vi "TxData_Organization_EVM_Selection_EIRP_only.vi"() -> ()   [LabVIEW 2023, in "ParsingData.lvlib"]
uses:
  <vilib>/Utility/file.llb/Read Delimited Spreadsheet (string).vi
  <vilib>/Utility/file.llb/Read Delimited Spreadsheet (DBL).vi
  ParsingData.lvlib
panel:
  in  "EVM?":dbl=-30.0 format="%#_13g"
  in  "EIRP_res":dbl=10.0
  in  "EIRP_Max":dbl=60.0
  in  "EIRP_Min":dbl=-10.0
  in  "CalPower ¸ÉÀv":dbl=70.0 format="%#_13g"
  in  "Input power_res":dbl=5.0
  in  "Input power_up":dbl=-20.0
  in  "Input power_low":dbl=-60.0
  out "Maximum_EIRP":T1 caption="Maximum EIRP"
  out "Minimum_EIRP":T1 caption="Minimum EIRP"
  out "Best EVM with EIRP steps":T2(array[cluster])
  in  "File Path":path=path "D:/_Project/_Code/LabVIEW/L_og_Backup/Cindy_20250224_litepoint_UD0630_one_panel"
  out "Max EVM : Mode             Polarity                     UD att                BFIC COM att           BFIC ele att                SG Power                      EIRP                           EVM":string[](array[string])
  out "EVM to EIRP":cluster{dbl[], "all rows":dbl[]}[](graph)
  # "X:EIRP        Y:EVM"
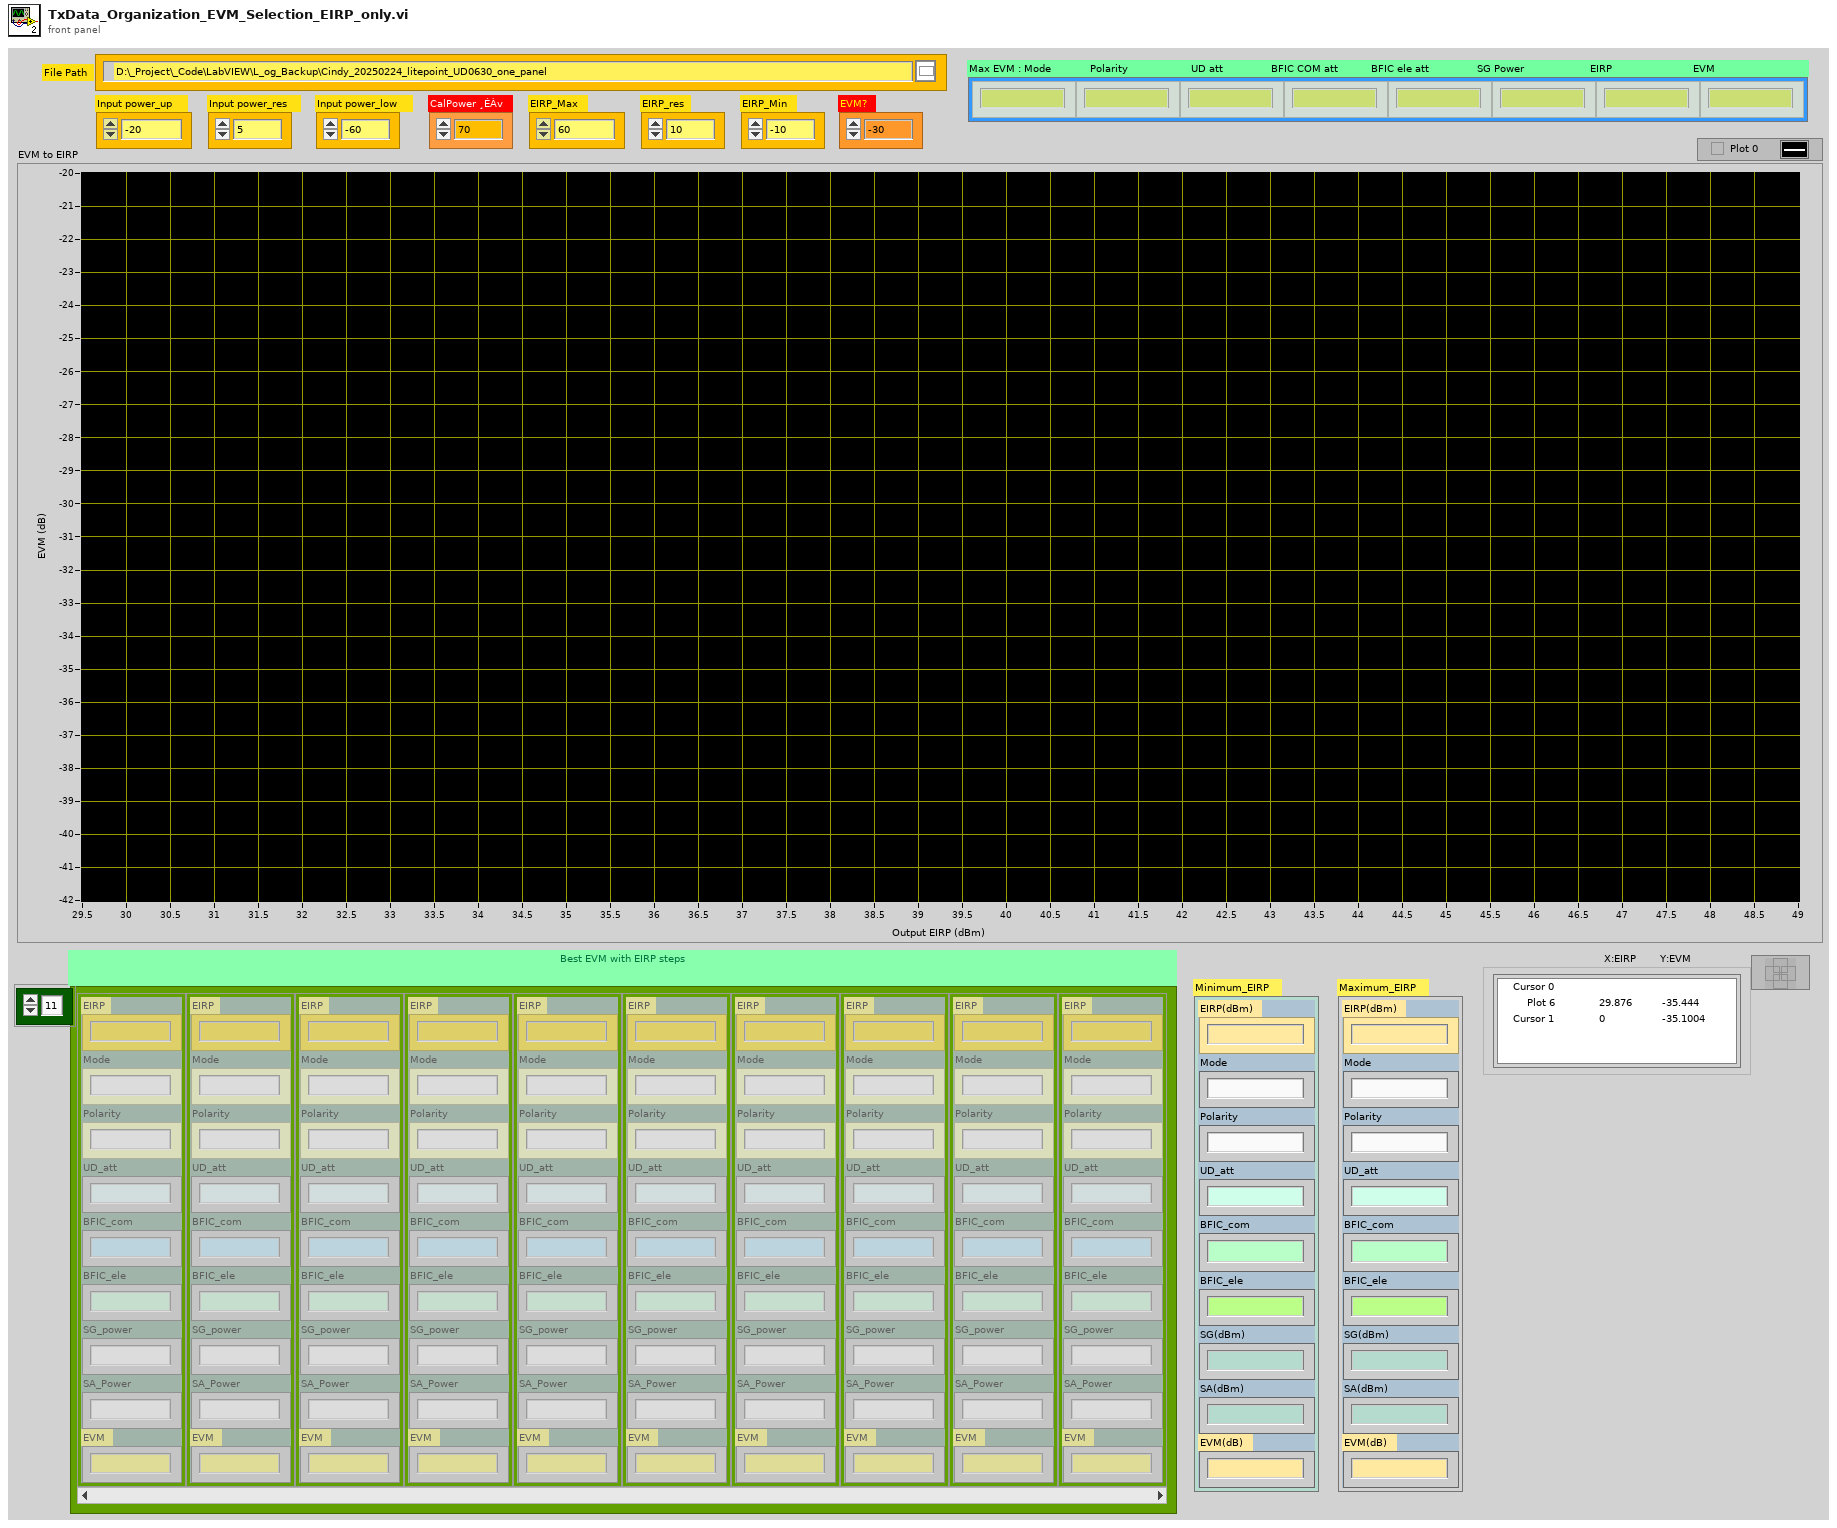
[diagram p1: front panel]
types:
  T1 = cluster{"EIRP(dBm)":string, "Mode":string, "Polarity":string, "UD_att":string, "BFIC_com":string, "BFIC_ele":string, "SG(dBm)":string, "SA(dBm)":string, "EVM(dB)":string}
  T2 = cluster{"EIRP":string, "Mode":string, "Polarity":string, "UD_att":string, "BFIC_com":string, "BFIC_ele":string, "SG_power":string, "SA_Power":string, "EVM":string}[]
  T3 = cluster{"[0]":string, "[1]":string, "[2]":string, "[3]":string, "[4]":string, "[5]":string, "[6]":string, "[7]":string, "[8]":string}
  T4 = cluster{"[0]":string, "[1]":string, "[2]":string, "[3]":string, "[4]":string, "[5]":string, "[6]":string, "[7]":string, "[8]":string}[]
  T5 = cluster{"EIRP":string, "Mode":string, "Polarity":string, "UD_att":string, "BFIC_com":string, "BFIC_ele":string, "SG_power":string, "SA_Power":string, "EVM":string}
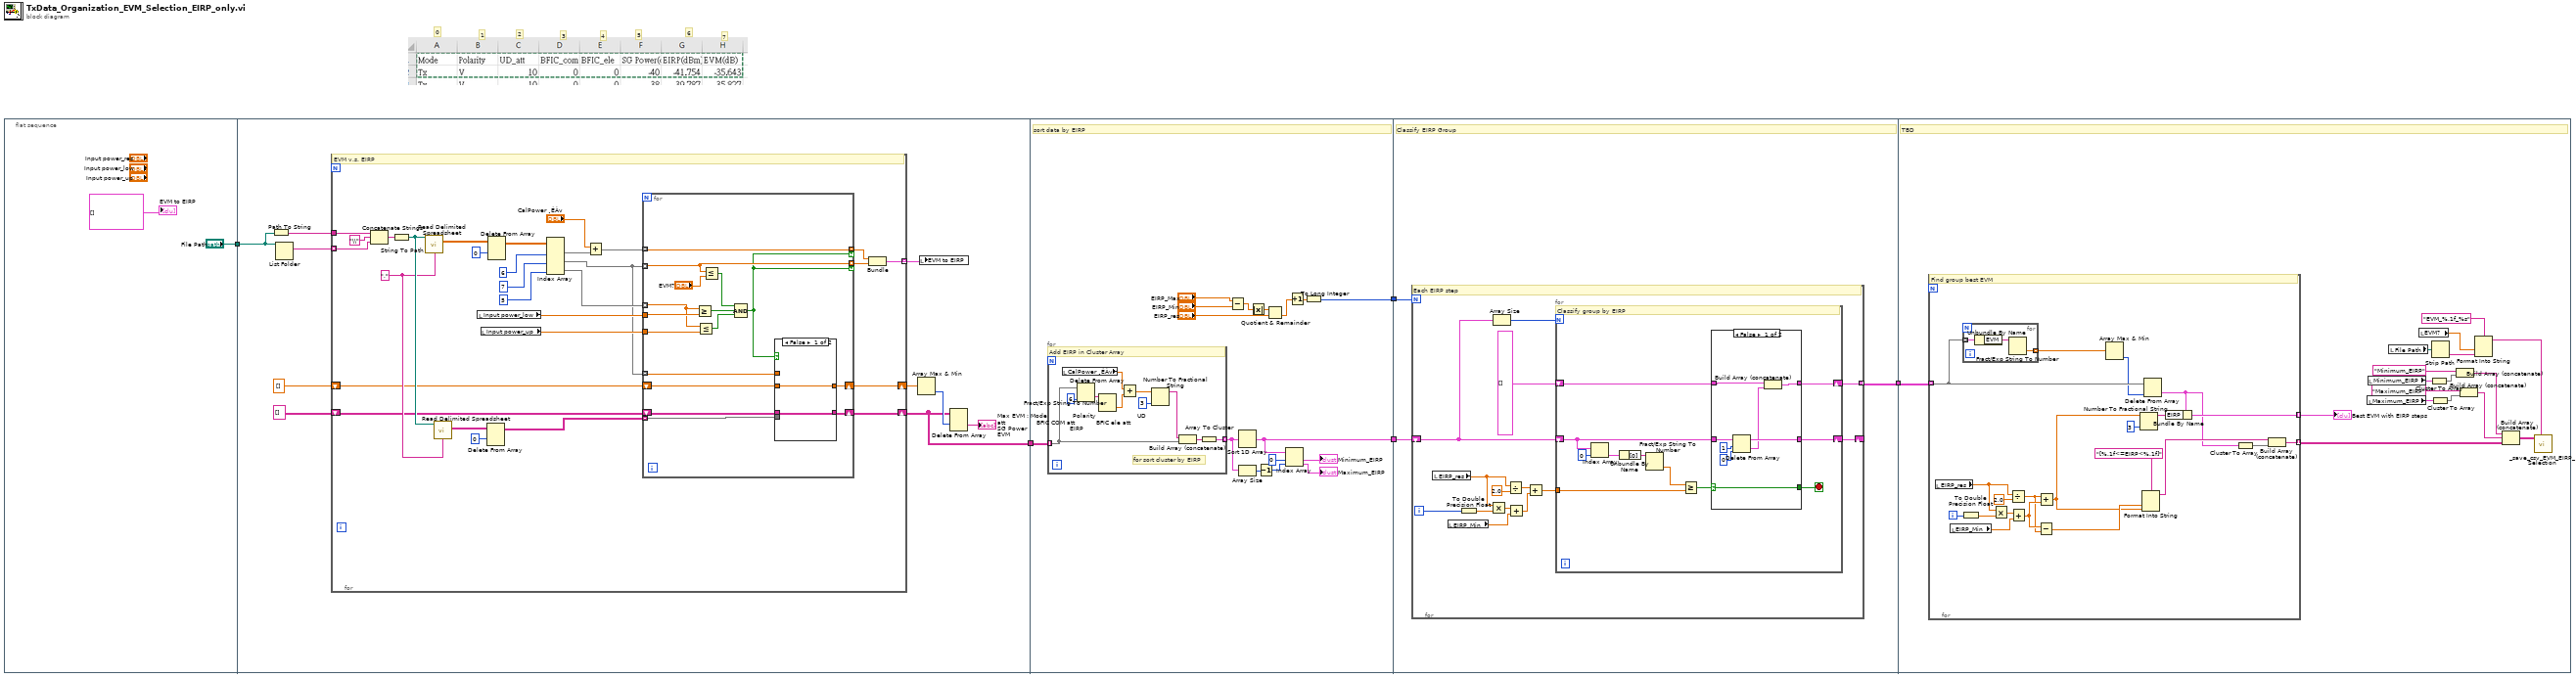
[diagram p0: block diagram]
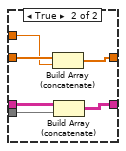
[diagram p2: hidden frame]
diagram:
  # "7"
  # "6"
  # "5"
  # "4"
  # "3"
  # "2"
  # "1"
  # "0"
  n1 = flat-sequence {
    tunnel: ["File Path"] -> w5
    tunnel: [w8] -> w1
    tunnel: w5 -> [w11]
    tunnel: w1 -> [w78]
    tunnel: [w76] -> w4
    tunnel: [w82] -> w3
    tunnel: w4 -> [w98]
    tunnel: w3 -> [w99]
    tunnel: [w97] -> w2
    tunnel: w2 -> [w152]
    frame #0 {
      "EVM to EIRP" <- cluster{dbl[], dbl[]}[] []
    }
    frame #1 {
      n2 = Path To String(path=w11) -> (string=w16:string)
      n3 = List Folder(path=w11) -> (filenames=w17:string[])  [unwired: 3 in, 3 out]
      n4 = for {
        tunnel: w17 -> [w44] mode=indexing
        tunnel: w16 -> [w46]
        tunnel: [w36] -> w9 mode=indexing
        shift-right: [w18] -> w8
        shift-left: string[][] [] -> [w22]
        shift-right: [w19] -> w14
        shift-left: dbl[] [] -> [w23]
        w27 = "," ("delimiter (\\t)")
        # "EVM v.s. EIRP"
        n5 = Concatenate Strings(w46, "\\" ("string"), w44) -> (w45:string)
        n6 = String To Path(string=w45) -> (path=w28:path)
        n7 = call-poly <vilib>:"Read Delimited Spreadsheet.vi"("file path (dialog if empty)"=w28, "delimiter (\\t)"=w27) -> ("all rows"=w42:dbl[][])  [unwired: 8 in, 5 out]
        n8 = call-poly <vilib>:"Read Delimited Spreadsheet.vi"("file path (dialog if empty)"=w28, "delimiter (\\t)"=w27) -> ("all rows"=w29:string[][])  [unwired: 8 in, 5 out]
        n9 = local read "Input power_low"() -> (w25:dbl)
        n10 = local read "Input power_up"() -> (w24:dbl)
        n11 = Delete From Array(array=w29, index (row)=0 ("disabled index (col)")) -> (array with subset deleted=w20:string[][])  [unwired: 2 in, 1 out]
        n12 = Delete From Array(array=w42, index (row)=0 ("disabled index (col)")) -> (array with subset deleted=w40:dbl[][])  [unwired: 2 in, 1 out]
        n13 = Index Array(array=w40, index (col) #1=6 ("disabled index (col)"), index (col) #2=7 ("index (col)"), index (col) #3=5 ("index (col)")) -> (element #1=w26:dbl[], element #2=w21:dbl[], element #3=w31:dbl[])  [unwired: 3 in]
        n14 = Add(x="CalPower ¸ÉÀv", y=w26) -> (x+y=w35:dbl[])
        n15 = for {
          tunnel: w35 -> [w60] mode=indexing
          tunnel: w21 -> [w61] mode=indexing
          tunnel: [w61] -> w33 mode=indexing if=w47
          tunnel: [w60] -> w34 mode=indexing if=w47
          tunnel: w31 -> [w58] mode=indexing
          tunnel: w25 -> [w59]
          tunnel: w24 -> [w57]
          shift-right: [w48] -> w19
          shift-left: w23 -> [w53]
          shift-right: [w49] -> w18
          shift-left: w22 -> [w51]
          tunnel: w21 -> [w52] mode=indexing
          tunnel: w20 -> [w50] mode=indexing
          n16 = Greater Or Equal?(x=w58, y=w59) -> (x >= y?=w55:bool)
          n17 = Less Or Equal?(x=w58, y=w57) -> (x <= y?=w56:bool)
          n18 = Less Or Equal?(x=w61, y="EVM?") -> (x <= y?=w54:bool)
          n19 = Compound Arithmetic op=AND(w54, w55, w56) -> (w47:bool)
          n20 = case shown="False" w47 {
            tunnel: w53 -> [w64 w70]
            tunnel: w52 -> [_ w69]
            tunnel: w51 -> [w63 w68]
            tunnel: w50 -> [_ w67]
            tunnel: [w63 w66] -> w49
            tunnel: [w64 w65] -> w48
            frame False {
            }
            frame True {
              n21 = Build Array (concatenate)(w70, w69) -> (w65:dbl[])
              n22 = Build Array (concatenate)(w68, w67) -> (w66:string[][])
            }
          }
        }
        n23 = Bundle(w34, w33) -> (w36:cluster{dbl[], dbl[]})  [unwired: 1 in]
      }
      n24 = Array Max & Min(array=w14) -> (min index (indices)=w13:i32)  [unwired: 3 out]
      n25 = local write "EVM to EIRP"(w9) -> ()
      n26 = Delete From Array(array=w8, index (row)=w13) -> (deleted portion=→"Max EVM : Mode             Polarity                     UD att                BFIC COM att           BFIC ele att                SG Power                      EIRP                           EVM":string[])  [unwired: 2 in, 1 out]
    }
    frame #2 {
      # "sort data by EIRP"
      n27 = for {
        tunnel: w78 -> [w87] mode=indexing
        tunnel: [w96] -> w77 mode=indexing
        # "for sort cluster by EIRP"
        # "Add EIRP in Cluster Array"
        n28 = local read "CalPower ¸ÉÀv"() -> (w90:dbl)
        n29 = Delete From Array(array=w87, index=6) -> (deleted portion=w93:string)  [unwired: 1 in, 1 out]
        n30 = Fract/Exp String To Number(string=w93) -> (number=w91:dbl)  [unwired: 3 in, 1 out]
        n31 = Add(x=w90, y=w91) -> (x+y=w92:dbl)
        n32 = Number To Fractional String(number=w92, precision (6)=i16 3) -> (F-format string=w89:string)  [unwired: 2 in]
        n33 = Build Array (concatenate)(w89, w87) -> (w94:string[])
        n34 = Array To Cluster(array=w94) -> (cluster=w96:T3)
      }
      n35 = Subtract(x="EIRP_Max", y="EIRP_Min") -> (x-y=w86:dbl)
      n36 = Sort 1D Array(array=w77) -> (sorted array=w76:T4)
      n37 = Array Size(array=w77) -> (size(s)=w75:i32)
      n38 = Absolute Value(x=w86) -> (abs(x)=w84:dbl)
      n39 = Decrement(x=w75) -> (x-1=w74:i32)
      n40 = Quotient & Remainder(x=w84, y="EIRP_res") -> (floor(x/y)=w85:dbl)  [unwired: 1 out]
      n41 = Index Array(array=w76, index #1=0 ("index"), index #2=w74) -> (element #1=→"Minimum_EIRP":T3, element #2=→"Maximum_EIRP":T3)
      n42 = Increment(x=w85) -> (x+1=w83:dbl)
      n43 = To Long Integer(number=w83) -> (32bit integer=w82:i32)
    }
    frame #3 {
      # "Classify EIRP Group"
      n44 = for {
        N: w99 -> [_]
        shift-right: [w104] -> _
        shift-left: w98 -> [w101]
        tunnel: [w103] -> w97 mode=indexing
        i -> [w109]
        # "Each EIRP step"
        n45 = local read "EIRP_res"() -> (w108:dbl)
        n46 = local read "EIRP_Min"() -> (w106:dbl)
        n47 = To Double Precision Float(number=w109) -> (double precision float=w107:dbl)
        n48 = Multiply(x=w108, y=w107) -> (x*y=w111:dbl)
        n49 = Array Size(array=w101) -> (size(s)=w102:i32)
        n50 = Divide(x=w108, y=2.0) -> (x/y=w112:dbl)
        n51 = Add(x=w111, y=w106) -> (x+y=w113:dbl)
        n52 = Add(x=w112, y=w113) -> (x+y=w105:dbl)
        n53 = for {
          N: w102 -> [_]
          tunnel: w105 -> [w120]
          shift-right: [w114] -> w104
          shift-left: w101 -> [w118]
          shift-right: [w116] -> w103
          shift-left: T2 [] ("reversed array") -> [w117]
          stop <- w115 stop-if-true
          # "Classify group by EIRP"
          n54 = Index Array(array=w118, index=0) -> (element=w124:T3)
          n55 = Unbundle By Name(w124) -> ("[0]"=w121:string)
          n56 = Fract/Exp String To Number(string=w121) -> (number=w122:dbl)  [unwired: 3 in, 1 out]
          n57 = Greater Or Equal?(x=w122, y=w120) -> (x >= y?=w119:bool)
          n58 = case shown="False" w119 {
            selector: w119 -> [w128 w135]
            tunnel: [w128 w135] -> w115
            tunnel: w118 -> [w132 w134]
            tunnel: [w129 w134] -> w114
            tunnel: w117 -> [w127 w133]
            tunnel: [w126 w133] -> w116
            frame False {
              n59 = Delete From Array(array=w132, length=1, index=0) -> (deleted portion=w125:T4, array with subset deleted=w129:T4)
              n60 = Build Array (concatenate)(w127, w125) -> (w126:T4)
            }
            frame True {
            }
          }
        }
      }
    }
    frame #4 {
      # "TBD"
      n61 = for {
        tunnel: w152 -> [w172] mode=indexing
        tunnel: [w154] -> w151 mode=indexing
        tunnel: [w167] -> w148 mode=indexing
        i -> [w161]
        # "Find group best EVM"
        n62 = local read "EIRP_res"() -> (w164:dbl)
        n63 = local read "EIRP_Min"() -> (w166:dbl)
        n64 = To Double Precision Float(number=w161) -> (double precision float=w165:dbl)
        n65 = for {
          tunnel: w172 -> [w176] mode=indexing
          tunnel: [w174] -> w173 mode=indexing
          n66 = Unbundle By Name(w176) -> ("EVM"=w175:string)
          n67 = Fract/Exp String To Number(string=w175) -> (number=w174:dbl)  [unwired: 3 in, 1 out]
        }
        n68 = Multiply(x=w164, y=w165) -> (x*y=w162:dbl)
        n69 = Divide(x=w164, y=2.0) -> (x/y=w159:dbl)
        n70 = Add(x=w162, y=w166) -> (x+y=w160:dbl)
        n71 = Subtract(x=w160, y=w159) -> (x-y=w157:dbl)
        n72 = Add(x=w159, y=w160) -> (x+y=w155:dbl)
        n73 = Array Max & Min(array=w173) -> (min index (indices)=w171:i32)  [unwired: 3 out]
        n74 = Number To Fractional String(number=w155, precision (6)=i16 3) -> (F-format string=w168:string)  [unwired: 2 in]
        n75 = Format Into String(format string="[%.1f<=EIRP<%.1f]", w157, w155) -> (resulting string=w156:string)  [unwired: 2 in, 1 out]
        n76 = Delete From Array(array=w172, index=w171) -> (deleted portion=w153:T5)  [unwired: 1 in, 1 out]
        n77 = Bundle By Name(cluster=w153, "EIRP"=w168) -> (w154:T5)
        n78 = Cluster To Array(cluster=w153) -> (array=w169:string[])
        n79 = Build Array (concatenate)(w156, w169) -> (w167:string[])
      }
      "Best EVM with EIRP steps" <- w151
      n80 = local read "Maximum_EIRP"() -> (w143:T1)
      n81 = local read "Minimum_EIRP"() -> (w146:T1)
      n82 = local read "File Path"() -> (w150:path)
      n83 = local read "EVM?"() -> (w138:dbl)
      n84 = Cluster To Array(cluster=w146) -> (array=w145:string[])
      n85 = Strip Path(path=w150) -> (name=w137:string)  [unwired: 1 out]
      n86 = Cluster To Array(cluster=w143) -> (array=w142:string[])
      n87 = Build Array (concatenate)("Minimum_EIRP" ("format string"), w145) -> (w140:string[])
      n88 = Build Array (concatenate)("Maximum_EIRP" ("format string"), w142) -> (w141:string[])
      n89 = Format Into String(format string="EVM_%.1f_%s", w138, w137) -> (resulting string=w136:string)  [unwired: 2 in, 1 out]
      n90 = Build Array (concatenate)(w140, w141, w148) -> (w149:string[][])
      n91 = call "_save_csv_EVM_EIRP_Selection.vi"("NoteName"=w136, "array in"=w149) -> ()  [unwired: 9 in, 1 out]
    }
  }
